vi "Start Async.vi"(8 "error in (no error)":errorcluster, 11 "gRPC service in":refnum<class "Bus_Monitor_API.lvclass">) -> (0 "error out":errorcluster, 3 "gRPC service out":refnum<class "Bus_Monitor_API.lvclass">)   [LabVIEW 2025, in "bus_monitor_server.lvlib" / "Bus_Monitor_API.lvclass"]
uses:
  Bus_Monitor_API.lvclass
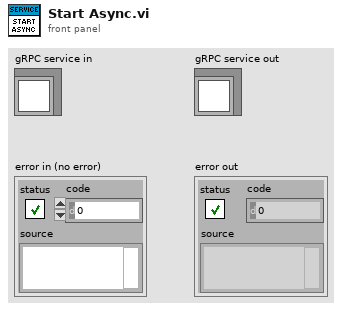
[diagram p1: front panel]
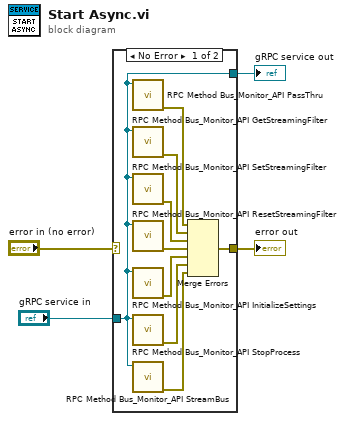
[diagram p0: block diagram]
diagram:
  n1 = case shown="No Error" "error in (no error)" {
    selector: "error in (no error)" -> [_ w15]
    tunnel: [w13 w15] -> w3
    tunnel: [w12 w14] -> w1
    tunnel: "gRPC service in" -> [w12 w14]
    frame No Error {
      n2 = call "RPC Method Bus_Monitor_API PassThru.vi"("gRPC service in"=w12) -> ("error out"=w11:errorcluster)  [unwired: 9 in, 1 out]
      n3 = call "RPC Method Bus_Monitor_API GetStreamingFilter.vi"("gRPC service in"=w12) -> ("error out"=w10:errorcluster)  [unwired: 9 in, 1 out]
      n4 = call "RPC Method Bus_Monitor_API SetStreamingFilter.vi"("gRPC service in"=w12) -> ("error out"=w9:errorcluster)  [unwired: 9 in, 1 out]
      n5 = call "RPC Method Bus_Monitor_API ResetStreamingFilter.vi"("gRPC service in"=w12) -> ("error out"=w8:errorcluster)  [unwired: 9 in, 1 out]
      n6 = call "RPC Method Bus_Monitor_API InitializeSettings.vi"("gRPC service in"=w12) -> ("error out"=w7:errorcluster)  [unwired: 9 in, 1 out]
      n7 = call "RPC Method Bus_Monitor_API StopProcess.vi"("gRPC service in"=w12) -> ("error out"=w6:errorcluster)  [unwired: 9 in, 1 out]
      n8 = call "RPC Method Bus_Monitor_API StreamBus.vi"("gRPC service in"=w12) -> ("error out"=w5:errorcluster)  [unwired: 9 in, 1 out]
      n9 = Merge Errors(w11, w10, w9, w8, w7, w6, w5) -> (w13:errorcluster)
    }
    frame Error {
    }
  }
  "error out" <- w3
  "gRPC service out" <- w1
